vi "Image Resize Example.vi"() -> ()   [LabVIEW 2020]
doc: "G-Image example demonstrating image resizing with various filters."
uses:
  Image Processing/Controls/Resize Filter.ctl
  <vilib>/picture/picture.llb/imagedata.ctl
  Image IO/Polymorphic VIs/Load Image (Path).vi
  G-Image.lvlib
panel:
  in  "Image Scale":dbl(slide)=1.0 min=0.1 max=5.0 step=0.1 scale=0.1..5.0
  in  "Image":u16(ring) items=["amiga-juggler.gif", "gradient.png", "LV5-about.png", "test-pattern.png", "vector-gradient.svg", "vector.svg"]
  in  "Stop":bool
  in  "Filter":T1
  out "2D Picture":picture
  # "Instructions:\n1. Run the VI.\n2. Select an image to resize from the Image ring.\n3. Adjust Image Scale to resize the image.\n4. Compare image quality with different Filter settings."
  # "G"
  # "-Image"
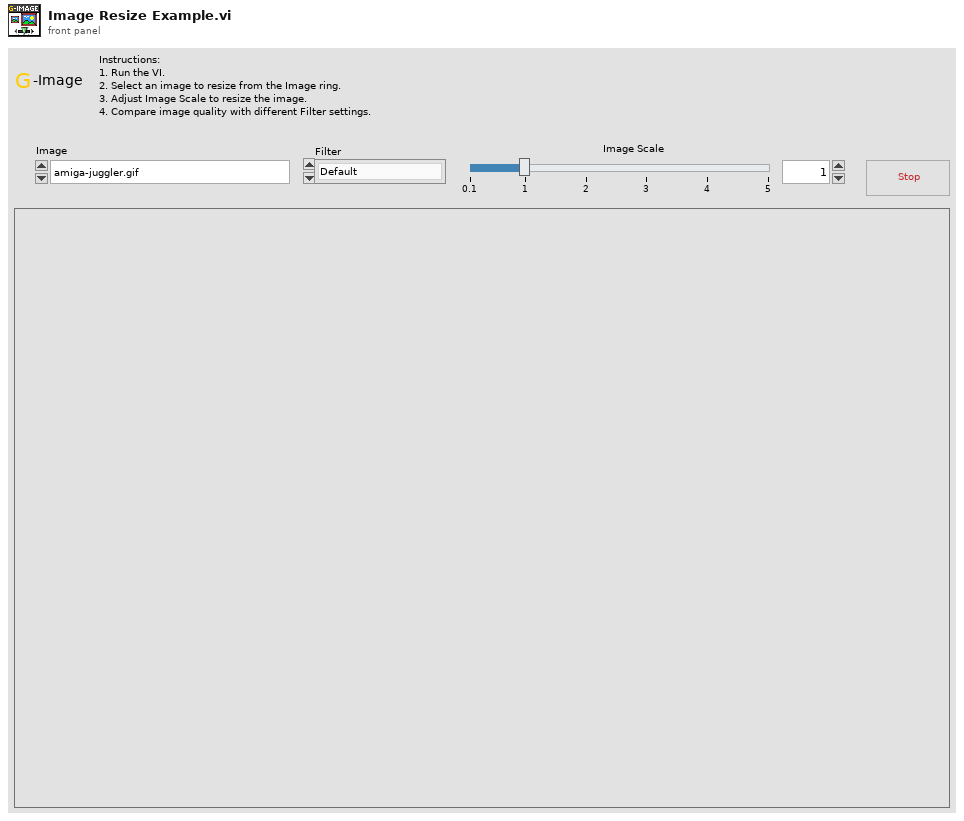
[diagram p1: front panel]
types:
  T1 = typedef "G-Image.lvlib/Resize Filter.ctl" = enum16{"Default", "Box", "Triangle", "Cubic B-Spline", "Catmull-Rom", "Mitchell"}
  T2 = typedef "imagedata.ctl" = cluster{"image type":i32, "image depth":i32, "image":u8[], "mask":u8[], "colors":u32[], "Rectangle":cluster{"left":i16, "top":i16, "right":i16, "bottom":i16}}
  T3 = cluster{"left":i16, "top":i16, "right":i16, "bottom":i16}
  T4 = cluster{"left":dbl, "top":dbl, "right":dbl, "bottom":dbl}
  T5 = cluster{"left":i32, "top":i32, "right":i32, "bottom":i32}
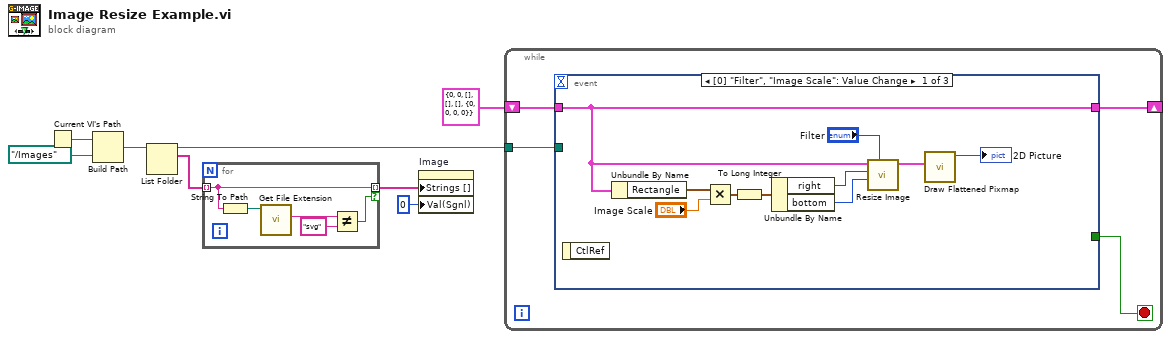
[diagram p0: block diagram]
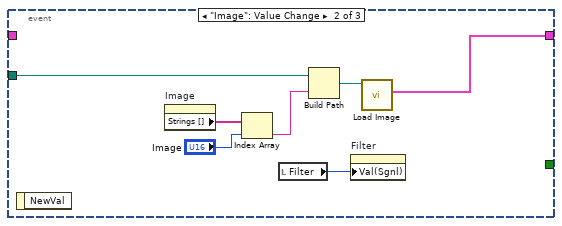
[diagram p2: hidden frame]
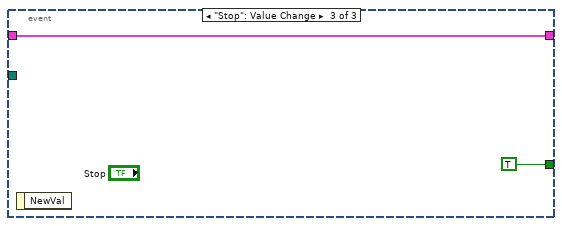
[diagram p3: hidden frame]
diagram:
  n1 = Current VI's Path() -> (path=w8:path)
  n2 = Build Path(base path=w8, name or relative path=path "../Images") -> (appended path=w6:path)
  n3 = List Folder(path=w6) -> (path out=w4:path, filenames=w2:string[])  [unwired: 3 in, 2 out]
  n4 = for {
    tunnel: w2 -> [w10] mode=indexing
    tunnel: [w10] -> w1 mode=indexing if=w9
    n5 = String To Path(string=w10) -> (path=w13:path)
    n6 = call <vilib>:"Get File Extension.vi"("file"=w13) -> ("lowercase file extension"=w12:string)  [unwired: 6 in, 4 out]
    n7 = Not Equal?(x=w12, y="svg") -> (x != y?=w9:bool)
  }
  n8 = property on="Image" class="Ring (strict)"("Strings []"=w1, "Val(Sgnl)"=u16 0 ("Value (Signaling)")) -> ()  [unwired: 2 in, 2 out]
  n9 = while {
    tunnel: w4 -> [w16]
    shift-right: [w15] -> _
    shift-left: T2 {"image type"=0, "image depth"=0, "image"=[], "mask"=[], "colors"=[], "Rectangle"={"left"=0, "top"=0, "right"=0, "bottom"=0}} ("Image") -> [w14]
    stop <- w17 stop-if-true
    n10 = event shown="[0] \"Filter\", \"Image Scale\": Value Change" {
      selector: _ -> [_ _ _]
      dyn-events: _ -> [_ _ _]
      timeout: _ -> [_ _ _]
      tunnel: w14 -> [w20 _ w35]
      tunnel: [_ _ TRUE] -> w17
      tunnel: w16 -> [_ w32 _]
      tunnel: [w20 w30 w35] -> w15
      event "Image Scale": Value Change {
        n11 = event-data() -> ()  [unwired: 1 in, 1 out]
        n12 = Unbundle By Name(w20) -> ("Rectangle"=w24:T3)
        n13 = Multiply(x=w24, y="Image Scale") -> (x*y=w23:T4)
        n14 = To Long Integer(number=w23) -> (32bit integer=w18:T5)
        n15 = Unbundle By Name(w18) -> ("right"=w22:i32, "bottom"=w21:i32)
        n16 = call "Resize Image.vi"("Filter (Default)"="Filter", "Height"=w21, "Width"=w22, "Image"=w20) -> ("Resized Image"=w26:T2)  [unwired: 6 in, 1 out]
        n17 = call <vilib>:"Draw Flattened Pixmap.vi"("image data"=w26) -> ("new picture"=→"2D Picture":picture)  [unwired: 8 in]
      }
      event "Image": Value Change {
        n18 = event-data() -> ()  [unwired: 1 in, 1 out]
        n19 = property on="Image" class="Ring (strict)"() -> ("Strings []"=w34:string[])  [unwired: 2 in, 2 out]
        n20 = Index Array(array=w34, index="Image") -> (element=w33:string)
        n21 = local read "Filter"() -> (w29:T1)
        n22 = Build Path(base path=w32, name or relative path=w33) -> (appended path=w31:path)
        n23 = property on="Filter" class="Enum (strict)"("Val(Sgnl)"=w29) -> ()  [unwired: 2 in, 2 out]
        n24 = call-poly "Load Image.vi"("Path In"=w31) -> ("Image"=w30:T2)  [unwired: 8 in, 2 out]
      }
      event "Stop": Value Change {
        n25 = event-data() -> ()  [unwired: 1 in, 1 out]
      }
    }
  }
